vi "GPIO Read Value.vi"(7 "GPIO #":T1=-1, 8 "error in (no error)":errorcluster, 11 "FirmwareComms in":refnum<class "DeviceComms.lvclass">) -> (0 "error out":errorcluster, 2 "Value":bool, 3 "FirmwareComms out":refnum<class "DeviceComms.lvclass">)   [LabVIEW 2024, in "CTI.lvlib" / "DeviceComms.lvclass"]
uses:
  DeviceComms.lvclass
  GPIO Number.ctl
  CTI.lvlib
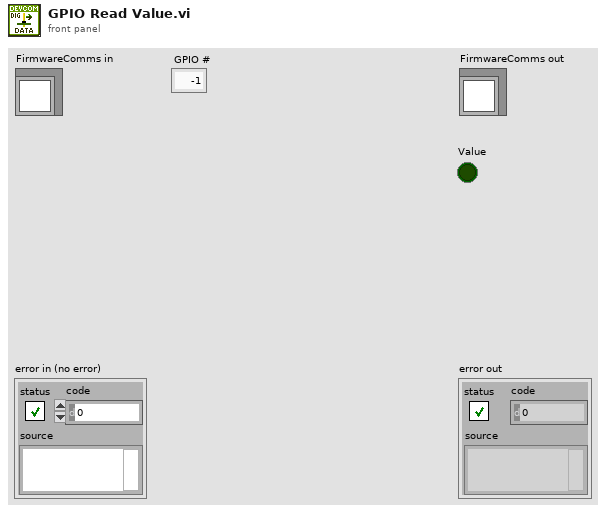
[diagram p1: front panel]
types:
  T1 = typedef "CTI.lvlib/GPIO Number.ctl" = i8
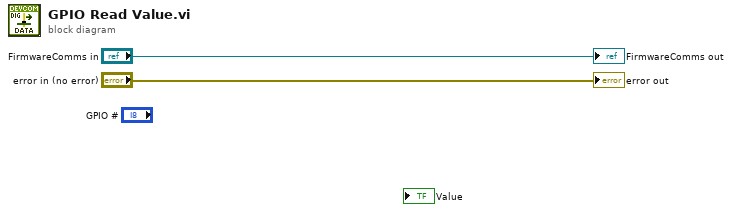
[diagram p0: block diagram]
diagram:
  "error out" <- "error in (no error)"
  "FirmwareComms out" <- "FirmwareComms in"
